vi "Encoder Filter.vi"(6 "Initialise":bool, 7 "Filter Iterations":i16=2, 9 "Pulse B":bool, 10 "Pulse A":bool) -> (1 "Filtered Pulse B":bool, 2 "Filtered Pulse A":bool)   [LabVIEW 2014]
doc: "Input pulse levels have to persist\nfor the number of filter iterations\nor they will be ignored.\nDR 25-10-2011"
uses:
  <vilib>/rvi/Emulation/niFpgaGetClockAttributes.vi
  <vilib>/rvi/Emulation/niFpgaSctlEmulationGetInTimedLoop.vi
  <vilib>/rvi/Emulation/niFpgaEmulationReportErrorSimple.vi
  <vilib>/rvi/Emulation/niFpgaCriticalErrorInLSC.vi
panel:
  # "Input pulse levels have to persist\nfor the number of filter iterations\nor they will be ignored."
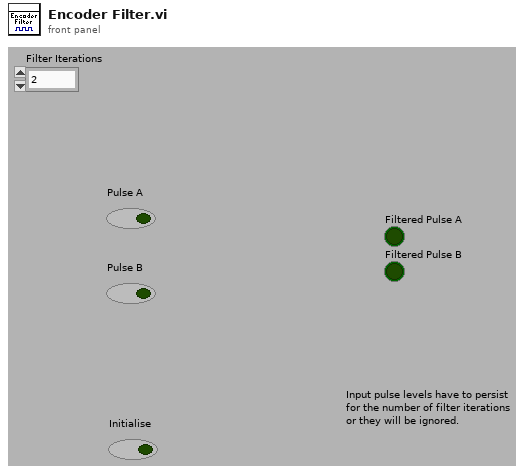
[diagram p1: front panel]
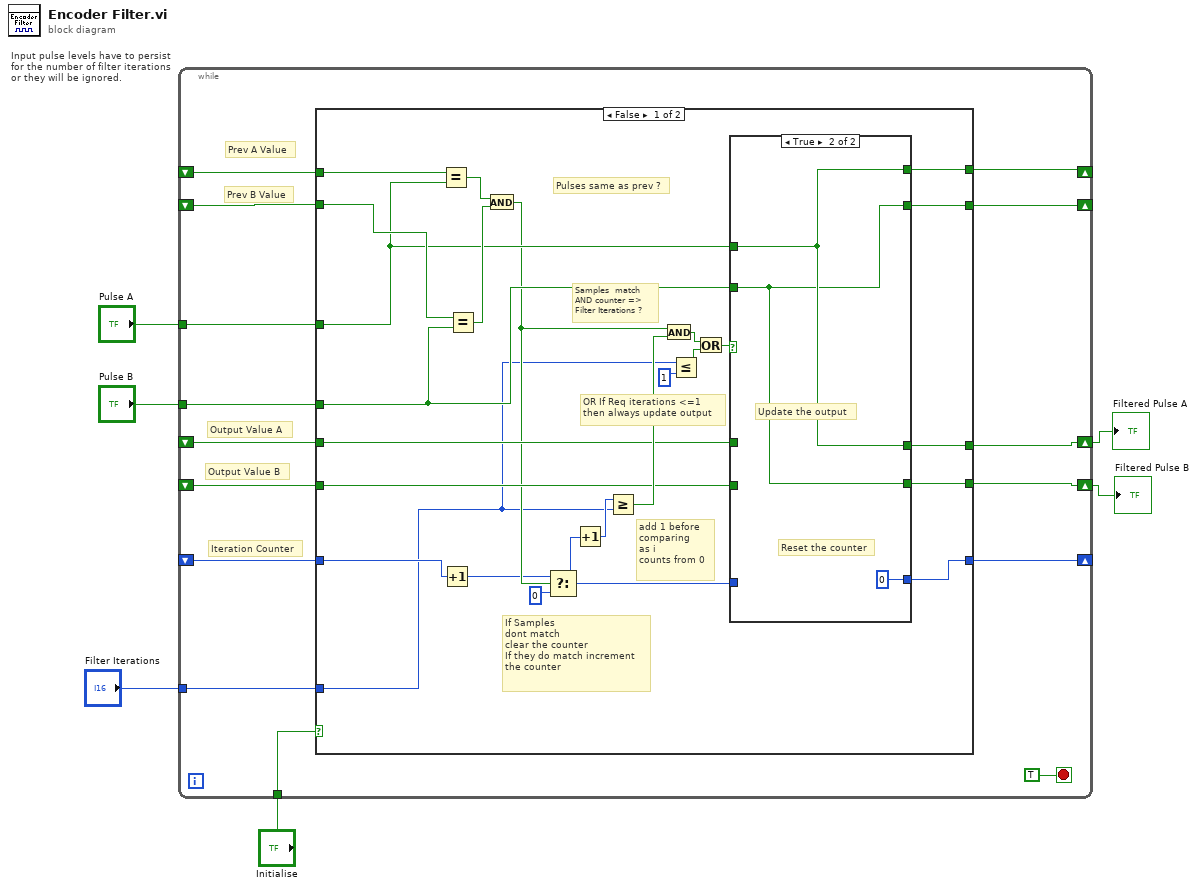
[diagram p0: block diagram]
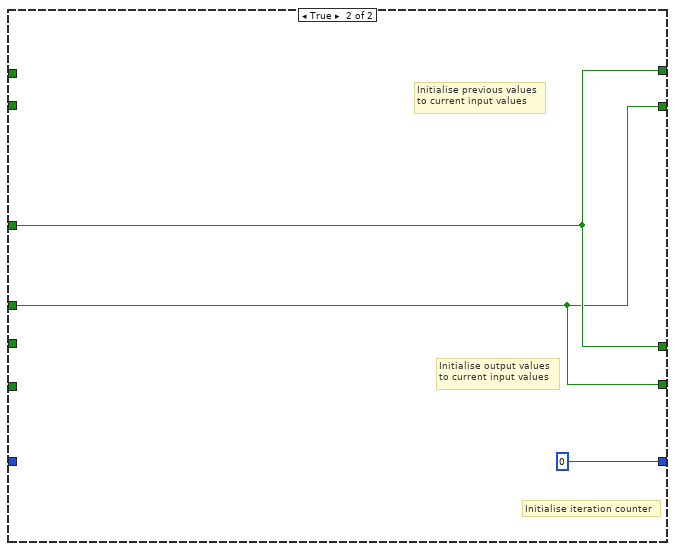
[diagram p3: hidden frame]
diagram:
  # "Input pulse levels have to persist\nfor the number of filter iterations\nor they will be ignored."
  n1 = while {
    tunnel: "Initialise" -> [w21]
    shift-right: [w20] -> _
    shift-left: _ -> [w19]
    shift-right: [w16] -> w2
    shift-left: _ -> [w14]
    shift-right: [w15] -> w1
    shift-left: _ -> [w13]
    tunnel: "Pulse A" -> [w18]
    tunnel: "Pulse B" -> [w17]
    shift-right: [w12] -> _
    shift-left: _ -> [w9]
    shift-right: [w11] -> _
    shift-left: _ -> [w10]
    tunnel: "Filter Iterations" -> [w8]
    stop <- TRUE stop-if-true
    # "Prev B Value"
    # "Prev A Value"
    # "Output Value B"
    # "Output Value A"
    # "Iteration Counter"
    n2 = case shown="False" w21 {
      tunnel: [w41 i16 0] -> w20
      tunnel: w19 -> [w29 _]
      tunnel: w18 -> [w36 w56]
      tunnel: w17 -> [w35 w55]
      tunnel: [w38 w56] -> w16
      tunnel: [w37 w55] -> w15
      tunnel: w14 -> [w34 _]
      tunnel: w13 -> [w33 _]
      tunnel: [w43 w56] -> w12
      tunnel: [w42 w55] -> w11
      tunnel: w10 -> [w39 _]
      tunnel: w9 -> [w40 _]
      tunnel: w8 -> [w23 _]
      frame False {
        # "OR If Req iterations <=1\nthen always update output"
        # "add 1 before\ncomparing\nas i\ncounts from 0"
        # "Samples  match\nAND counter =>\nFilter Iterations ?"
        # "If Samples\ndont match\nclear the counter\nIf they do match increment\nthe counter"
        # "Pulses same as prev ?"
        n3 = Equal?(x=w40, y=w36) -> (x = y?=w46:bool)
        n4 = Increment(x=w29) -> (x+1=w30:i16)
        n5 = Equal?(x=w39, y=w35) -> (x = y?=w45:bool)
        n6 = And(x=w46, y=w45) -> (x .and. y?=w31:bool)
        n7 = Select(t=w30, s=w31, f=i16 0 ("Filter Iterations")) -> (s? t:f=w28:i16)
        n8 = Increment(x=w28) -> (x+1=w27:i16)
        n9 = Greater Or Equal?(x=w27, y=w23) -> (x >= y?=w44:bool)
        n10 = And(x=w31, y=w44) -> (x .and. y?=w26:bool)
        n11 = Less Or Equal?(x=w23, y=i16 1 ("Filter Iterations")) -> (x <= y?=w24:bool)
        n12 = Or(x=w26, y=w24) -> (x .or. y?=w25:bool)
        n13 = case shown="True" w25 {
          tunnel: [w48 w53] -> w43
          tunnel: [w47 w52] -> w42
          tunnel: w28 -> [w51 _]
          tunnel: [w51 i16 0] -> w41
          tunnel: [w50 w53] -> w38
          tunnel: [w49 w52] -> w37
          tunnel: w36 -> [w48 w53]
          tunnel: w35 -> [w47 w52]
          tunnel: w34 -> [w50 _]
          tunnel: w33 -> [w49 _]
          frame False {
            # "Don't\nlet output change"
          }
          frame True {
            # "Reset the counter"
            # "Update the output"
          }
        }
      }
      frame True {
        # "Initialise previous values\nto current input values"
        # "Initialise iteration counter"
        # "Initialise output values\nto current input values"
      }
    }
  }
  "Filtered Pulse A" <- w2
  "Filtered Pulse B" <- w1
